vi "Hatch Detect Reversed.vi"(7 "error in":errorcluster) -> (27 "error out":errorcluster)   [LabVIEW 2018]
uses:
  <vilib>/vision/driver/IMAQdx.llb/IMAQdx Camera Control Mode.ctl
  <vilib>/userdefined/High Color/IMAQdx.ctl
  <vilib>/vision/NI_Vision_Development_Module.lvlib
  <vilib>/vision/driver/NI_Vision_Acquisition_Software.lvlib
  <resource>/objmgr/imaqdx.rc
panel:
  in  "stop":bool
  in  "error in 2":errorcluster
  out "Image Out":T1(plugin-control)
types:
  T1 = typedef "IMAQ Image.ctl" = refnum<image>
  T2 = typedef "IMAQdx.ctl" = refnum<k21>
  T3 = typedef "NI_Vision_Acquisition_Software.lvlib/IMAQdx Camera Control Mode.ctl" = enum32{"Controller", "Listener"}
  T4 = typedef "Image Type" = u32
  T5 = cluster{"Measurement Parameter":i32, "Range Lower Value":dbl, "Range Upper Value":dbl, "Range":bool, "Measurement Type":bool}[]
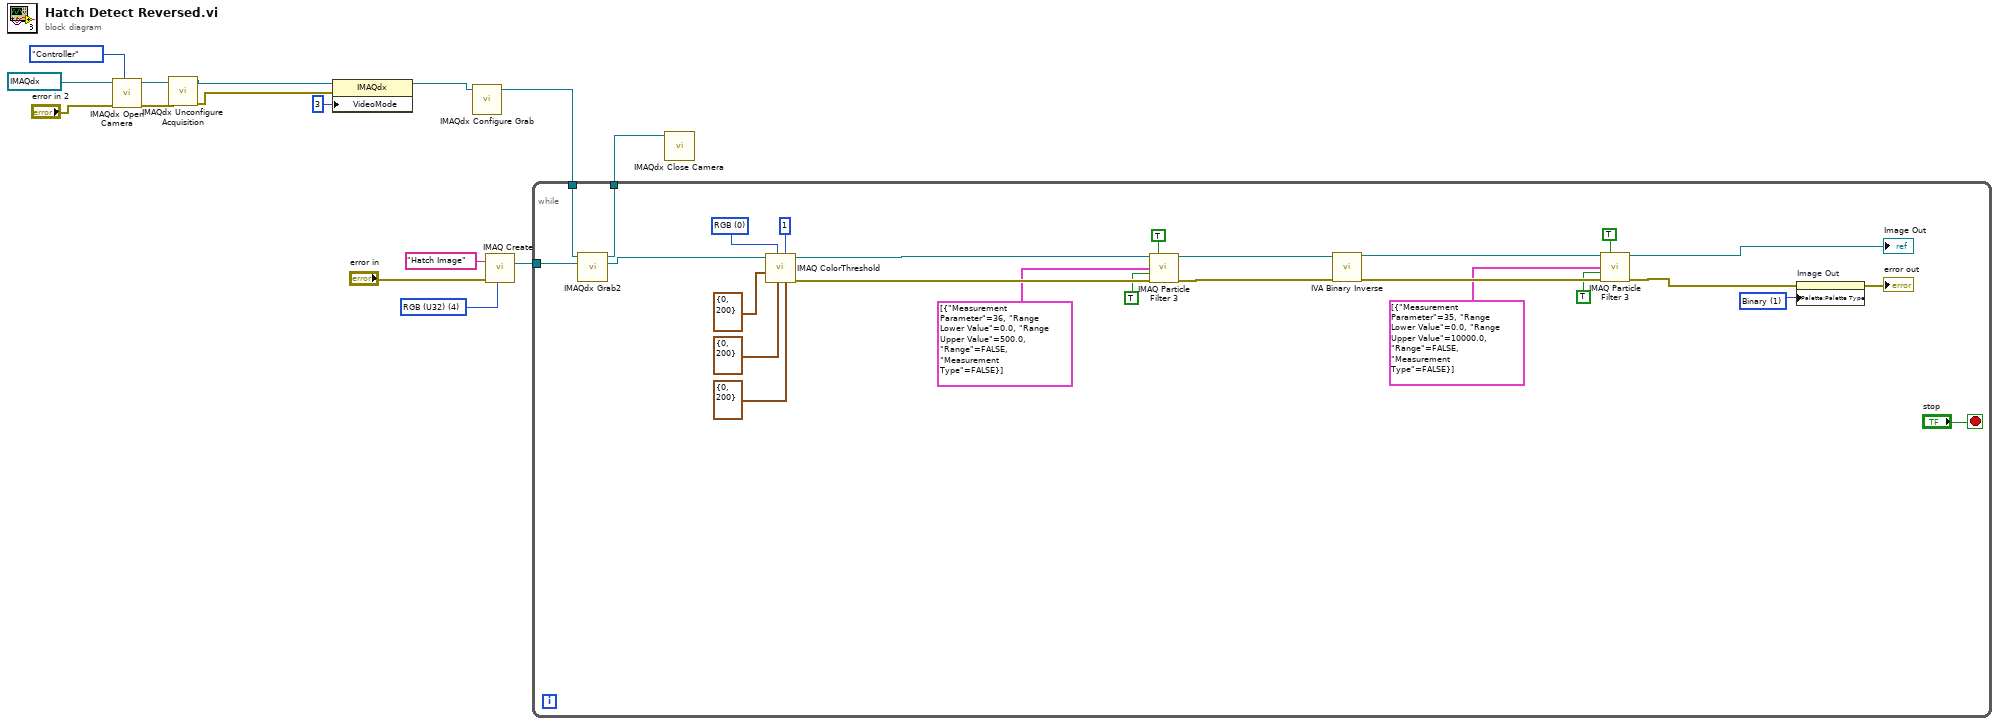
[diagram p0: block diagram]
diagram:
  w14 = T4 4 items=["Grayscale (U8)", "Grayscale (I16)", "Grayscale (SGL)", "Complex (CSG)", "RGB (U32)", "HSL (U32)", "RGB (U64)", "Grayscale (U16)"] ("Image Type")
  n1 = call <vilib>:"IMAQdx Open Camera.vi"("Camera Control Mode"=IMAQdx_Camera_Control_Mode."Controller", "error in"="error in 2", "Session In"=T2 "cam1") -> ("error out"=w8:errorcluster, "Session Out"=w7:T2)  [unwired: 7 in]
  n2 = call <vilib>:"IMAQdx Unconfigure Acquisition.vi"("error in"=w8, "Session In"=w7) -> ("error out"=w5:errorcluster, "Session Out"=w6:T2)  [unwired: 8 in]
  n3 = property class="IMAQdx"(reference=w6, error in=w5, "VideoMode"=u32 3) -> (reference out=w9:T2)  [unwired: 1 out]
  n4 = call <vilib>:"IMAQdx Configure Grab.vi"("Session In"=w9) -> ("Session Out"=w2:T2)  [unwired: 9 in, 1 out]
  n5 = call "IMAQ Create"("Image Name"="Hatch Image", "Image Type"=w14, "error in (no error)"="error in") -> ("New Image"=w4:T1)  [unwired: 1 in, 2 out]
  n6 = while {
    tunnel: w4 -> [w20]
    tunnel: w2 -> [w18]
    tunnel: [w17] -> w1
    stop <- "stop" stop-if-true
    w21 = u32 1 items=["Grayscale", "Binary", "Gradient", "Rainbow", "Temperature", "User Defined", "Binary 16 Bit", "Gradient 16 Bit", "Rainbow 16 Bit", "Temperature 16 Bit", "User Defined 16 Bit"] ("Palette Type")
    w40 = u16 0 items=["RGB", "HSL", "HSV", "HSI"] ("Color Mode")
    n7 = call <vilib>:"IMAQdx Grab2.vi"("Image In"=w20, "Session In"=w18) -> ("Image Out"=w19:T1, "Session Out"=w17:T2)  [unwired: 6 in, 2 out]
    n8 = call "IMAQ ColorThreshold"("Blue or Luma or Val or Inten Range"=cluster{"Lower value":i32, "Upper value":i32} {"Lower value"=0, "Upper value"=200}, "Replace Value"=1, "Green or Sat Range"=cluster{"Lower value":i32, "Upper value":i32} {"Lower value"=0, "Upper value"=200}, "Color Mode"=w40, "Red or Hue Range"=cluster{"Lower value":i32, "Upper value":i32} {"Lower value"=0, "Upper value"=200}, "Image Src"=w19) -> ("error out"=w36:errorcluster, "Image Dst Out"=w32:T1)  [unwired: 2 in, 2 out]
    n9 = call "IMAQ Particle Filter 3"("Image Src"=w32, "Connectivity 4/8 (8)"=TRUE, "Selection Values"=T5 [{"Measurement Parameter"=36, "Range Lower Value"=0.0, "Range Upper Value"=500.0, "Range"=FALSE, "Measurement Type"=FALSE}], "Keep/Remove Particles (F)"=TRUE ("Keep/Remove Particles"), "error in (no error)"=w36) -> ("Image Dst Out"=w30:T1, "error out"=w33:errorcluster)  [unwired: 4 in, 5 out]
    n10 = call <vilib>:"IVA Binary Inverse.vi"("error in (no error)"=w33, "Image In"=w30) -> ("error out"=w29:errorcluster, "Image Out"=w25:T1)  [unwired: 8 out]
    n11 = call "IMAQ Particle Filter 3"("Image Src"=w25, "Connectivity 4/8 (8)"=TRUE, "Selection Values"=T5 [{"Measurement Parameter"=35, "Range Lower Value"=0.0, "Range Upper Value"=10000.0, "Range"=FALSE, "Measurement Type"=FALSE}], "Keep/Remove Particles (F)"=TRUE ("Keep/Remove Particles"), "error in (no error)"=w29) -> ("Image Dst Out"=→"Image Out":T1, "error out"=w26:errorcluster)  [unwired: 4 in, 5 out]
    n12 = property on="Image Out" class="ImageControl"(error in=w26, "Palette:Palette Type"=w21) -> (error out=→"error out":errorcluster)  [unwired: 1 in, 1 out]
  }
  n13 = call <vilib>:"IMAQdx Close Camera.vi"("Session In"=w1) -> ()  [unwired: 10 in, 1 out]
